vi "MNK_TC to PGSQL.vi"(8 "error in (no error)":errorcluster, 9 "calibration string":string, 10 "description string":string, 11 "dbl":dbl[](array[numeric])) -> (0 "error out":errorcluster)   [LabVIEW 2013]
uses:
  postgreSQL-lv/Data.PG/Data.PGSQL.lvclass
panel:
  # "MNK TC to PGSQL"
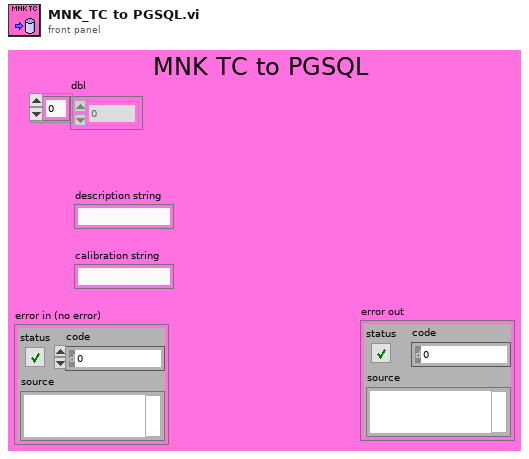
[diagram p1: front panel]
types:
  T1 = cluster{"dbl":dbl[], "description string":string, "calibration string":string}
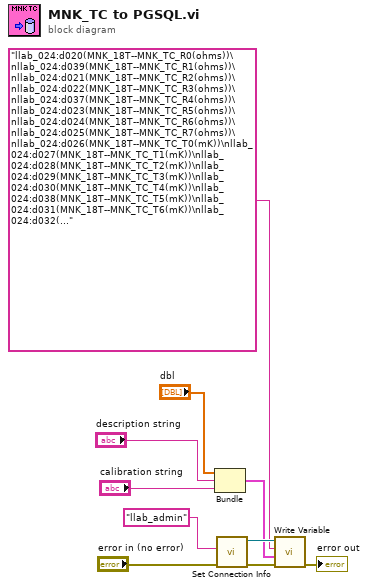
[diagram p0: block diagram]
diagram:
  n1 = Bundle("dbl"="dbl", "description string"="description string", "calibration string"="calibration string") -> (w7:T1)  [unwired: 1 in]
  n2 = call "Set Connection Info.vi"("username"="llab_admin", "error in (no error)"="error in (no error)") -> ("Data.PG out"=w10:refnum<class "Data.PGSQL.lvclass">, "error out"=w9:errorcluster)  [unwired: 7 in]
  n3 = call "Write Variable.vi"("error in (no error)"=w9, "Data"=w7, "variable"="llab_024:d020(MNK_18T--MNK_TC_R0(ohms))\nllab_024:d039(MNK_18T--MNK_TC_R1(ohms))\nllab_024:d021(MNK_18T--MNK_TC_R2(ohms))\nllab_024:d022(MNK_18T--MNK_TC_R3(ohms))\nllab_024:d037(MNK_18T--MNK_TC_R4(ohms))\nllab_024:d023(MNK_18T--MNK_TC_R5(ohms))\nllab_024:d024(MNK_18T--MNK_TC_R6(ohms))\nllab_024:d025(MNK_18T--MNK_TC_R7(ohms))\nllab_024:d026(MNK_18T--MNK_TC_T0(mK))\nllab_024:d027(MNK_18T--MNK_TC_T1(mK))\nllab_024:d028(MNK_18T--MNK_TC_T2(mK))\nllab_024:d029(MNK_18T--MNK_TC_T3(mK))\nllab_024:d030(MNK_18T--MNK_TC_T4(mK))\nllab_024:d038(MNK_18T--MNK_TC_T5(mK))\nllab_024:d031(MNK_18T--MNK_TC_T6(mK))\nllab_024:d032(MNK_18T--MNK_TC_T7(mK))\nllab_024:d033(MNK_18T--MNK_TC_I0(Amp))\nllab_024:d034(MNK_18T--MNK_TC_I1(Amp))\nllab_024:d035(MNK_18T--MNK_TC_I2(Amp))\nllab_024:d036(MNK_18T--MNK_TC_I3(Amp))", "Data.PG in"=w10) -> ("error out"=→"error out":errorcluster)  [unwired: 5 in, 2 out]
